vi "Sha-1.vi"(1 "Message In as Byte Array":u8[](array[numeric])=[97, 98, 99, 100, 101, 102, 103, 104, 98, 99, 100, 101, 102, 103, 104, 105, 99, 100, 101, 102, 103, 104, 105, 106, 100, 101, 102, 103, 104, 105, 106, 107, 101, 102, 103, 104, 105, 106, 107, 108, 102, 103, 104, 105, 106, 107, 108, 109, 103, 104, 105, 106, 107, 108, 109, 110, 104, 105, 106, 107, 108, 109, 110, 111, 105, 106, 107, 108, 109, 110, 111, 112, 106, 107, 108, 109, 110, 111, 112, 113, 107, 108, 109, 110, 111, 112, 113, 114, 108, 109, 110, 111, 112, 113, 114, 115, 109, 110, 111, 112, 113, 114, 115, 116, 110, 111, 112, 113, 114, 115, 116, 117]) -> (0 "Digest":u8[](array[numeric]) format="%x")   [LabVIEW 2014]
panel:
  # "Refactor Note:\n\nNeed to change inputs and outputs from\nstring to byte arrays"
  # "Test Vector:\n\n448 Bits:\nabcdbcdecdefdefgefghfghighijhijkijkljklmklmnlmnomnopnopq\n\nExpected Output In Hex:\n84983e44 1c3bd26e baae4aa1 f95129e5 e54670f1\n\n896 Bits:\nabcdefghbcdefghicdefghijdefghijkefghijklfghijklmghijklmnhijklmnoijklmnopjklmnopqklmnopqrlmnopqrsmnopqrstnopqrstu\n\nExpect Output In Hex:\na49b2446 a02c645b f419f995 b6709125 3a04a259"
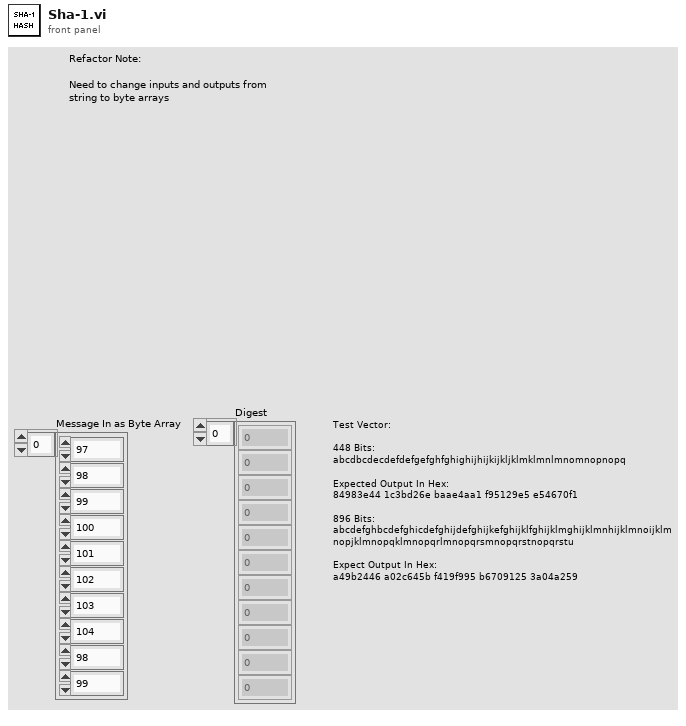
[diagram p1: front panel]
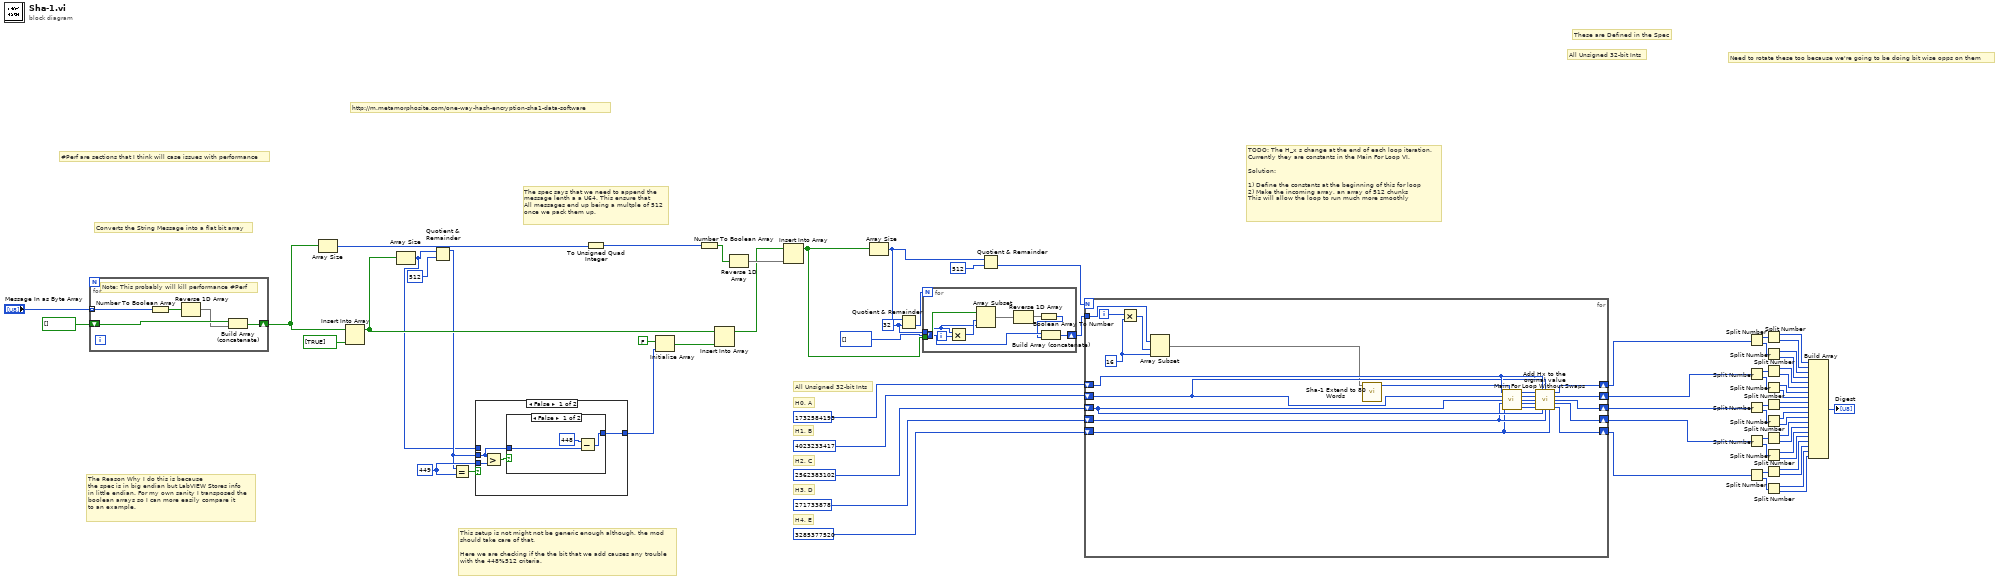
[diagram p0: block diagram]
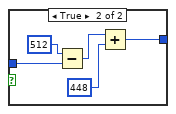
[diagram p2: hidden frame]
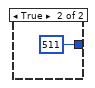
[diagram p3: hidden frame]
diagram:
  w3 = 32 ("y")
  w61 = 449 ("y")
  # "All Unsigned 32-bit Ints"
  # "H0, A"
  # "H3, D"
  # "H4, E"
  # "H2, C"
  # "H1, B"
  # "TODO: The H_x s change at the end of each loop iteration. \nCurrently they are constants in the Main For Loop VI. \n\nSolution:\n\n1) Define the constants at the beginning of this for loop\n2) Make the incoming array, an array of 512 chunks\nThis will allow the loop to run much more smoothly"
  # "These are Defined in the Spec"
  # "Need to rotate these too because we're going to be doing bit wise opps on them"
  # "#Perf are sections that I think will case issues with performance"
  # "The spec says that we need to append the\nmessage lenth a a U64. This ensure that \nAll messages end up being a multple of 512\nonce we pack them up."
  # "This setup is not might not be generic enough although, the mod\nshould take care of that.\n\nHere we are checking if the the bit that we add causes any trouble\nwith the 448%512 criteria."
  # "Converts the String Message into a flat bit array"
  # "The Reason Why I do this is because\nthe spec is in big endian but LabVIEW Stores info\nin little endian. For my own sanity I transposed the \nboolean arrays so I can more easily compare it\nto an example."
  # "http://m.metamorphosite.com/one-way-hash-encryption-sha1-data-software"
  # "All Unsigned 32-bit Ints"
  n1 = for {
    tunnel: "Message In as Byte Array" -> [w72] mode=indexing
    shift-right: [w70] -> w55
    shift-left: bool[] [] -> [w69]
    # "Note: This probably will kill performance #Perf"
    n2 = Number To Boolean Array(number=w72) -> (Boolean array=w71:bool[])
    n3 = Reverse 1D Array(array=w71) -> (reversed array=w68:bool[])
    n4 = Build Array (concatenate)(w69, w68) -> (w70:bool[])
  }
  n5 = Array Size(array=w55) -> (size(s)=w53:i32)
  n6 = Insert Into Array(array=w55, new element=bool[] [TRUE]) -> (w64:bool[])  [unwired: 1 in]
  n7 = Array Size(array=w64) -> (size(s)=w54:i32)
  n8 = Quotient & Remainder(x=w54, y=512) -> (x-y*floor(x/y)=w60:i32)  [unwired: 1 out]
  n9 = Equal?(x=w60, y=w61) -> (x = y?=w62:bool)
  n10 = case shown="False" w62 {
    tunnel: [w74 511 ("y")] -> w59
    tunnel: w61 -> [w75 _]
    tunnel: w60 -> [w73 _]
    tunnel: w54 -> [_ _]
    frame False {
      n11 = Greater?(x=w73, y=w75) -> (0:w76:bool)
      n12 = case shown="False" w76 {
        tunnel: w73 -> [w79 w84]
        tunnel: [w77 w81] -> w74
        frame False {
          n13 = Subtract(x=448, y=w79) -> (x-y=w77:i32)
        }
        frame True {
          n14 = Subtract(x=512 ("y"), y=w84) -> (x-y=w83:i32)
          n15 = Add(x=w83, y=448) -> (x+y=w81:i32)
        }
      }
    }
    frame True {
    }
  }
  n16 = To Unsigned Quad Integer(1:w53) -> (0:w56:u64)
  n17 = Initialize Array(FALSE, w59) -> (w63:bool[])
  n18 = Number To Boolean Array(number=w56) -> (Boolean array=w51:bool[])
  n19 = Insert Into Array(array=w64, new element=w63) -> (w46:bool[])  [unwired: 1 in]
  n20 = Reverse 1D Array(array=w51) -> (reversed array=w52:bool[])
  n21 = Insert Into Array(array=w46, new element=w52) -> (w4:bool[])  [unwired: 1 in]
  n22 = Array Size(array=w4) -> (size(s)=w6:i32)
  n23 = Quotient & Remainder(x=w6, y=w3) -> (floor(x/y)=w5:i32)  [unwired: 1 out]
  n24 = for {
    N: w5 -> [_]
    tunnel: w4 -> [w94]
    tunnel: w3 -> [w90]
    shift-right: [w88] -> w1
    shift-left: u32[] [] -> [w87]
    i -> [w92]
    n25 = Multiply(x=w90, y=w92) -> (x*y=w91:i32)
    n26 = Array Subset(array=w94, index=w91, length=w90) -> (w93:bool[])
    n27 = Reverse 1D Array(array=w93) -> (reversed array=w89:bool[])
    n28 = Boolean Array To Number(Boolean array=w89) -> (number=w86:u32)
    n29 = Build Array (concatenate)(w87, w86) -> (w88:u32[])
  }
  n30 = Quotient & Remainder(x=w6, y=512) -> (floor(x/y)=w57:i32)  [unwired: 1 out]
  n31 = for {
    N: w57 -> [_]
    shift-right: [w110] -> w43
    shift-left: u32 1732584193 -> [w104]
    shift-right: [w109] -> w30
    shift-left: u32 4023233417 -> [w103]
    shift-right: [w108] -> w21
    shift-left: u32 2562383102 -> [w102]
    shift-right: [w107] -> w20
    shift-left: u32 271733878 -> [w101]
    shift-right: [w106] -> w17
    shift-left: u32 3285377520 -> [w100]
    tunnel: w1 -> [w96]
    i -> [w99]
    w98 = 16 ("length")
    n32 = Multiply(x=w99, y=w98) -> (x*y=w97:i32)
    n33 = Array Subset(array=w96, index=w97, length=w98) -> (w95:u32[])
    n34 = call "Sha-1 Extend to 80 Words.vi"("16 32-bit Words In"=w95) -> ("80 32 Bit Words Out"=w105:u32[])  [unwired: 10 in]
    n35 = call "Main For Loop Without Swaps.vi"("A"=w104, "80 32-bit Words"=w105, "B"=w103, "C"=w102, "D"=w101, "E"=w100) -> ("A Out"=w115:u32, "B Out"=w114:u32, "C Out"=w113:u32, "D Out"=w112:u32, "E Out"=w111:u32)  [unwired: 5 in]
    n36 = call "Add Hx to the orginal value.vi"("A Out"=w115, "H0 In"=w104, "H1 In"=w103, "B Out"=w114, "C Out"=w113, "D Out"=w112, "E Out"=w111, "H2 In"=w102, "H3 In"=w101, "H4 In"=w100) -> ("H0"=w110:u32, "H1"=w109:u32, "H2"=w108:u32, "H3"=w107:u32, "H4"=w106:u32)  [unwired: 1 in]
  }
  n37 = Split Number(x=w43) -> (hi(x)=w42:u16, lo(x)=w41:u16)
  n38 = Split Number(x=w30) -> (hi(x)=w35:u16, lo(x)=w36:u16)
  n39 = Split Number(x=w21) -> (hi(x)=w28:u16, lo(x)=w29:u16)
  n40 = Split Number(x=w20) -> (hi(x)=w22:u16, lo(x)=w23:u16)
  n41 = Split Number(x=w17) -> (hi(x)=w19:u16, lo(x)=w18:u16)
  n42 = Split Number(x=w42) -> (hi(x)=w40:u8, lo(x)=w39:u8)
  n43 = Split Number(x=w41) -> (hi(x)=w38:u8, lo(x)=w37:u8)
  n44 = Split Number(x=w35) -> (hi(x)=w34:u8, lo(x)=w33:u8)
  n45 = Split Number(x=w36) -> (hi(x)=w32:u8, lo(x)=w31:u8)
  n46 = Split Number(x=w28) -> (hi(x)=w27:u8, lo(x)=w26:u8)
  n47 = Split Number(x=w29) -> (hi(x)=w25:u8, lo(x)=w24:u8)
  n48 = Split Number(x=w22) -> (hi(x)=w16:u8, lo(x)=w15:u8)
  n49 = Split Number(x=w23) -> (hi(x)=w14:u8, lo(x)=w13:u8)
  n50 = Split Number(x=w19) -> (hi(x)=w12:u8, lo(x)=w11:u8)
  n51 = Split Number(x=w18) -> (hi(x)=w10:u8, lo(x)=w9:u8)
  n52 = Build Array(w40, w39, w38, w37, w34, w33, w32, w31, w27, w26, w25, w24, w16, w15, w14, w13, w12, w11, w10, w9) -> (→"Digest":u8[])
